vi "CryoServer GUI.vi"(9 "Standalone":bool=TRUE, 10 "Init Data":variant, 11 "Filter Wheel name":string) -> ()   [LabVIEW 2021]
uses:
  CryoServer cluster Settings.ctl
  CryoServer.lvclass
  CryoServer Telemetry Map.ctl
  Subsystems/SS typedef cluster Instrument Command Queue Data.ctl
  Subsystems/SS cluster Data Queue type.ctl
  CryoServer Channel Mapping.ctl
  hk-channel-class/HK Item/HK Channel cluster Telemetry Data.ctl
  hk-channel-class/HK Item/HK Channel enum Data Type.ctl
  <vilib>/Utility/error.llb/DialogType.ctl
  typedefs/CC cluster Alarm Data.ctl
  <vilib>/Analysis/baseanly.llb/Mean (DBL).vi
  hk-channel-class/HK Item/HK Item.lvclass
  <vilib>/Analysis/NI_AALBase.lvlib
panel:
  in  "Settings":bool
  in  "System Health":bool
  in  "HK Window":bool
  in  "Close":bool
  in  "Re-connect":bool
  in  "IP Address":string
  out "Response":string
  in  "Send":bool
  in  "Piper Board ID (Hex)":u32=10 format="%02x"
  in  "Piper Command":string
  out "Connected?":bool
  in  "Temperatures Values":i32[](listbox)
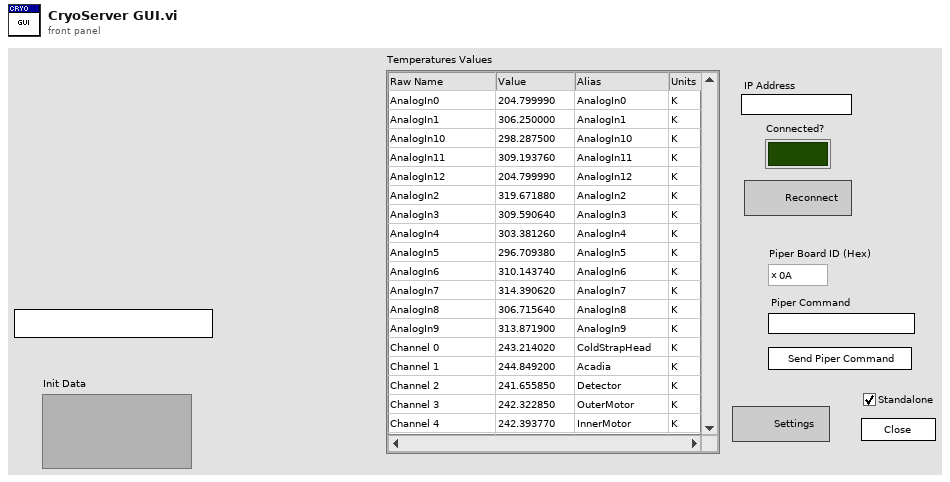
[diagram p1: front panel]
types:
  T1 = typedef "CryoServer cluster Settings.ctl" = cluster{"Address":string}
  T2 = typedef "CryoServer Telemetry Map.ctl" = map{string, dbl[]}
  T3 = typedef "SS typedef cluster Instrument Command Queue Data.ctl" = cluster{"Cmd":string, "Parameters":variant}
  T4 = typedef "CryoServer Channel Mapping.ctl" = cluster{"Alias":string, "Units":string}
  T5 = cluster{"state":refnum<user-event>, "Settings":T1, "CryoServer":refnum<class "CryoServer.lvclass">, "Telem":T2, "cntrl q":refnum<queue>, "Data Q":refnum<queue>, "Ch Names":string[], "Values":dbl[], "Cmd":T3, "Next Poll":timestamp, "error":errorcluster, "Ch Map":map{string, T4}, "Setting VI":refnum<vi>}
  T6 = typedef "SS cluster Data Queue type.ctl" = cluster{"Source":string, "Type":string, "Data":variant}
  T7 = typedef "HK Item.lvclass/HK Channel enum Data Type.ctl" = enum16{"Floating Point", "Integer", "Enum", "String", "Waveform", "File"}
  T8 = typedef "HK Item.lvclass/HK Channel cluster Telemetry Data.ctl" = cluster{"Ch Names":string[], "Ch Values":dbl[], "Timestamp":timestamp, "Data Type":T7}
  T9 = typedef "CC cluster Alarm Data.ctl" = cluster{"Measured Value":dbl, "Alarm Low":dbl, "Alarm High":dbl, "Message":string, "Source":string}
  T10 = typedef "DialogType.ctl" = u16
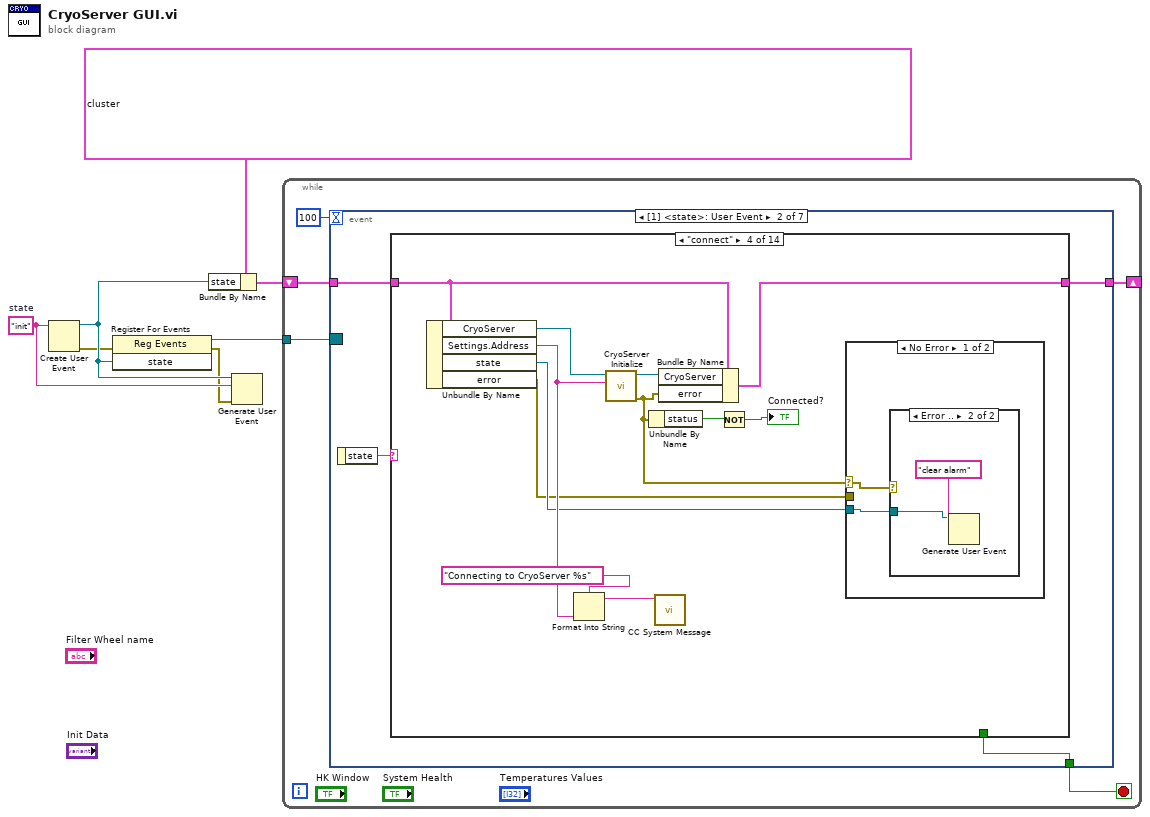
[diagram p0: block diagram]
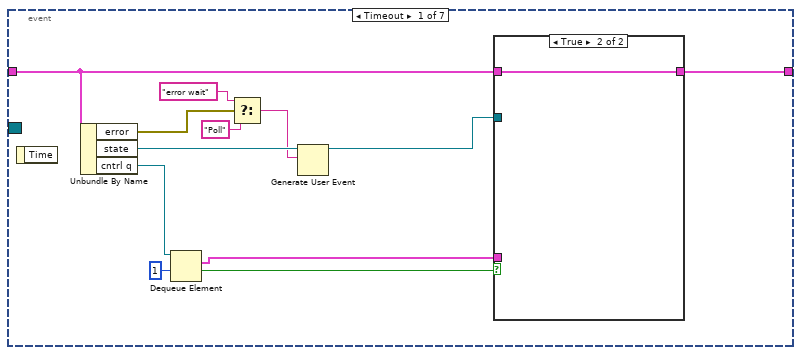
[diagram p2: hidden frame]
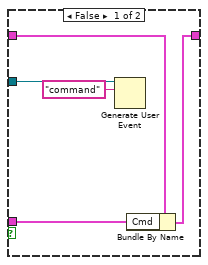
[diagram p3: hidden frame]
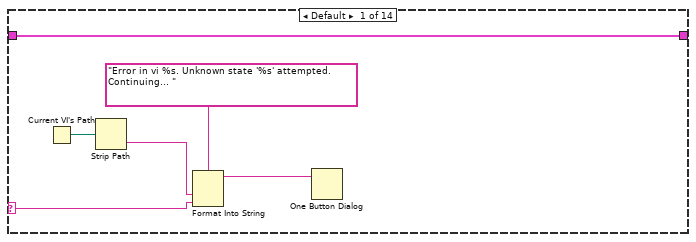
[diagram p4: hidden frame]
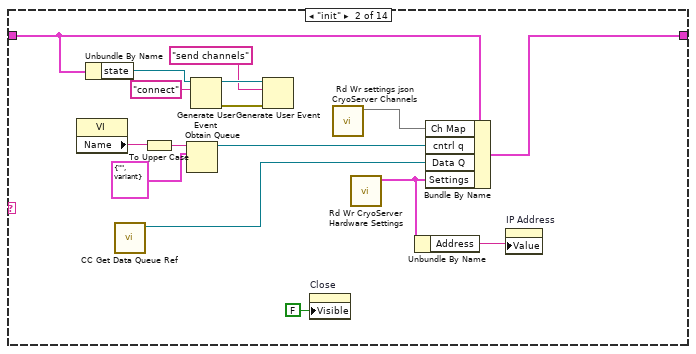
[diagram p5: hidden frame]
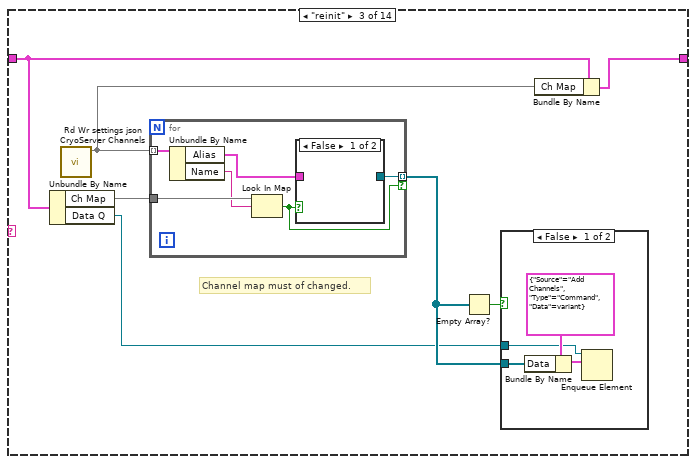
[diagram p6: hidden frame]
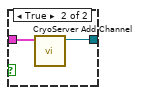
[diagram p8: hidden frame]
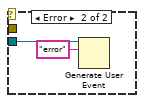
[diagram p10: hidden frame]
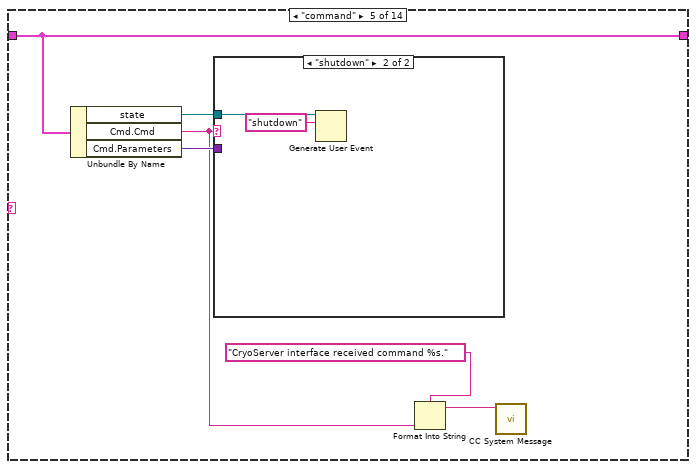
[diagram p11: hidden frame]
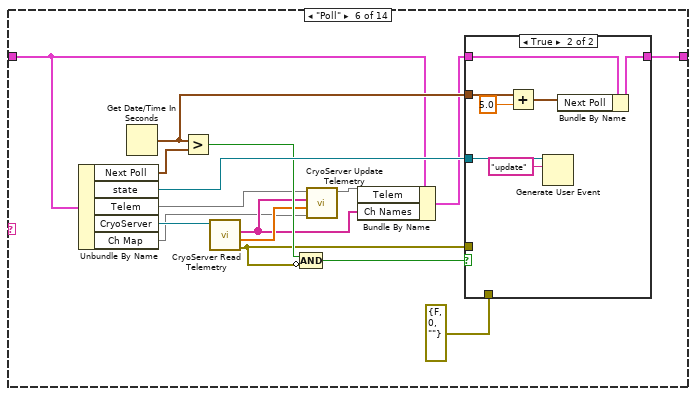
[diagram p13: hidden frame]
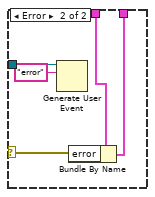
[diagram p15: hidden frame]
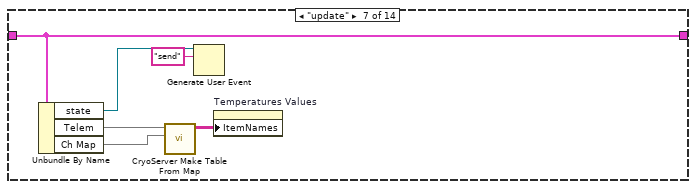
[diagram p16: hidden frame]
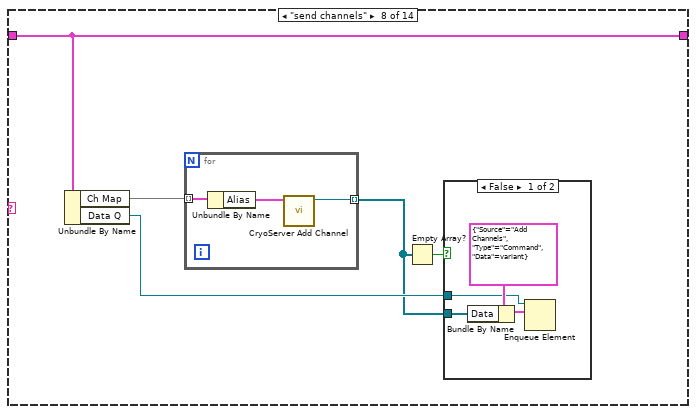
[diagram p17: hidden frame]
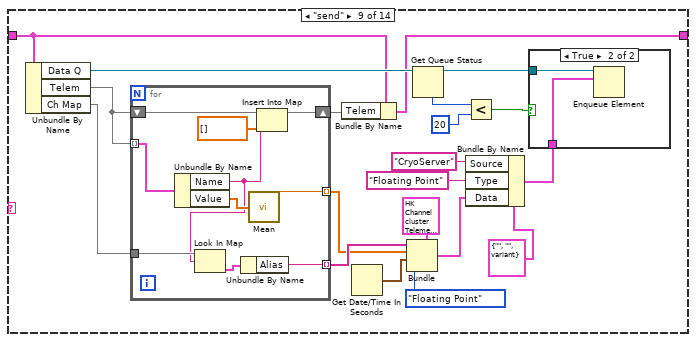
[diagram p19: hidden frame]
diagram:
  w3 = "init"  # state
  n1 = Create User Event(user event datatype=w3) -> (user event=w5:refnum<user-event>, error out=w1:errorcluster)  [unwired: 1 in]
  n2 = register-events(error in=w1, w5) -> (reference out=w4:refnum<event-registration>, error out=w2:errorcluster)  [unwired: 1 in]
  n3 = Bundle By Name(cluster=T5 {"state"=refnum, "Settings"={"Address"=""}, "CryoServer"=refnum, "Telem"={}, "cntrl q"=refnum, "Data Q"=refnum, "Ch Names"=[], "Values"=[], "Cmd"={"Cmd"="", "Parameters"=variant}, "Next Poll"=timestamp(0 s since 1904-01-01), "error"={"status"=FALSE, "code"=0, "source"=""}, "Ch Map"={}, "Setting VI"=refnum}, "state"=w5) -> (w6:T5)
  n4 = Generate User Event(user event=w5, event data cluster=w3, error in=w2) -> ()  [unwired: 1 in, 2 out]
  n5 = while {
    tunnel: w4 -> [w12]
    shift-right: [w10] -> _
    shift-left: w6 -> [w11]
    stop <- w9 stop-if-true
    n6 = event shown="[1] <state>: User Event" {
      selector: w12 -> [_ _ _ _ _ _ _]
      dyn-events: _ -> [_ _ _ _ _ _ _]
      timeout: 100 -> [_ _ _ _ _ _ _]
      tunnel: w11 -> [w17 w33 w239 w240 w251 w258 w261]
      tunnel: [w20 w32 w239 w241 w252 w258 w261] -> w10
      tunnel: [_ w31 _ _ _ _ _] -> w9
      event Timeout {
        n7 = event-data() -> ()  [unwired: 1 in, 1 out]
        n8 = Unbundle By Name(w17) -> ("error"=w16:errorcluster, "state"=w19:refnum<user-event>, "cntrl q"=w24:refnum<queue>)
        n9 = Dequeue Element(queue=w24, timeout in ms (-1)=1) -> (element=w21:T3, timed out?=w22:bool)  [unwired: 1 in, 2 out]
        n10 = Select(t="error wait" ("event data"), s=w16, f="Poll" ("event data")) -> (s? t:f=w13:string)
        n11 = Generate User Event(user event=w19, event data cluster=w13) -> (user event out=w18:refnum<user-event>)  [unwired: 2 in, 1 out]
        n12 = case shown="True" w22 {
          tunnel: w17 -> [w29 w30]
          tunnel: w21 -> [w28 _]
          tunnel: w18 -> [w27 _]
          tunnel: [w25 w30] -> w20
          frame False {
            n13 = Generate User Event(user event=w27, event data cluster="command" ("event data")) -> ()  [unwired: 2 in, 2 out]
            n14 = Bundle By Name(cluster=w29, "Cmd"=w28) -> (w25:T5)
          }
          frame True {
          }
        }
      }
      event User Event {
        n15 = event-data() -> ("state"=w34:string)  [unwired: 1 in]
        n16 = case shown="\"connect\"" w34 {
          selector: w34 -> [w39 _ _ _ _ _ _ _ _ _ _ _ _ _]
          tunnel: w33 -> [w35 w53 w62 w85 w99 w108 w138 w141 w154 w189 w194 w216 w219 w232]
          tunnel: [w35 w56 w63 w77 w99 w115 w138 w141 w155 w189 w199 w216 w219 w232] -> w32
          tunnel: [_ _ _ _ _ _ _ _ _ _ _ _ _ TRUE] -> w31
          frame Default {
            n17 = Current VI's Path() -> (path=w38:path)
            n18 = Strip Path(path=w38) -> (name=w37:string)  [unwired: 1 out]
            n19 = Format Into String(format string="Error in vi %s. Unknown state '%s' attempted. Continuing... ", w37, w39) -> (resulting string=w36:string)  [unwired: 2 in, 1 out]
            n20 = One Button Dialog(message=w36) -> ()  [unwired: 1 in, 1 out]
          }
          frame "init" {
            n21 = property class="VI"() -> ("Name"=w50:string)  [unwired: 2 in, 2 out]
            n22 = Unbundle By Name(w53) -> ("state"=w52:refnum<user-event>)
            n23 = call "CC Get Data Queue Ref.vi"() -> ("Data Q"=w46:refnum<queue>)  [unwired: 10 in, 1 out]
            n24 = To Upper Case(1:w50) -> (0:w49:string)
            n25 = Obtain Queue(name (unnamed)=w49, element data type=T3 {"Cmd"="", "Parameters"=variant}) -> (queue out=w47:refnum<queue>)  [unwired: 3 in, 2 out]
            n26 = Generate User Event(user event=w52, event data cluster="connect" ("event data")) -> (user event out=w44:refnum<user-event>, error out=w43:errorcluster)  [unwired: 2 in]
            n27 = Generate User Event(user event=w44, event data cluster="send channels" ("event data"), error in=w43) -> ()  [unwired: 1 in, 2 out]
            n28 = property on="Close" class="Bool"("Visible"=FALSE) -> ()  [unwired: 2 in, 2 out]
            n29 = call "Rd Wr settings json CryoServer Channels.vi"() -> ("CryoServer Channels out"=w45:map{string, T4})  [unwired: 9 in, 2 out]
            n30 = call "Rd Wr CryoServer Hardware Settings.vi"() -> ("CryoServer Settings"=w55:T1)  [unwired: 10 in, 1 out]
            n31 = Unbundle By Name(w55) -> ("Address"=w54:string)
            n32 = Bundle By Name(cluster=w53, "Ch Map"=w45, "cntrl q"=w47, "Data Q"=w46, "Settings"=w55) -> (w56:T5)
            n33 = property on="IP Address" class="Str"("Value"=w54) -> ()  [unwired: 2 in, 2 out]
          }
          frame "reinit" {
            # "Channel map must of changed."
            n34 = Unbundle By Name(w62) -> ("Ch Map"=w60:map{string, T4}, "Data Q"=w57:refnum<queue>)
            n35 = call "Rd Wr settings json CryoServer Channels.vi"() -> ("CryoServer Channels out"=w61:map{string, T4})  [unwired: 9 in, 2 out]
            n36 = for {
              tunnel: w61 -> [w72] mode=indexing
              tunnel: w60 -> [w73]
              tunnel: [w69] -> w58 mode=indexing if=w68
              n37 = Unbundle By Name(w72) -> ("Alias"=w70:T4, "Name"=w71:string)
              n38 = Look In Map(map=w73, key=w71) -> (key not found?=w68:bool)  [unwired: 1 in, 1 out]
              n39 = case shown="False" w68 {
                tunnel: w70 -> [_ w75]
                tunnel: [_ w74] -> w69
                frame False {
                }
                frame True {
                  n40 = call "CryoServer Add Channel.vi"("value"=w75) -> ("HK Item out"=w74:refnum<class "HK Item.lvclass">)  [unwired: 10 in]
                }
              }
            }
            n41 = Empty Array?(array=w58) -> (empty?=w59:bool)
            n42 = case shown="False" w59 {
              tunnel: w57 -> [w65 _]
              tunnel: w58 -> [w64 _]
              frame False {
                n43 = Bundle By Name(cluster=T6 {"Source"="Add Channels", "Type"="Command", "Data"=variant} ("element"), "Data"=w64) -> (w67:T6)
                n44 = Enqueue Element(queue=w65, element=w67) -> ()  [unwired: 2 in, 3 out]
              }
              frame True {
              }
            }
            n45 = Bundle By Name(cluster=w62, "Ch Map"=w61) -> (w63:T5)
          }
          frame "connect" {
            n46 = Unbundle By Name(w85) -> ("CryoServer"=w87:refnum<class "CryoServer.lvclass">, "Settings.Address"=w80:string, "state"=w78:refnum<user-event>, "error"=w76:errorcluster)
            n47 = Format Into String(format string="Connecting to CryoServer %s" ("Message"), w80) -> (resulting string=w81:string)  [unwired: 2 in, 1 out]
            n48 = call-dynamic "CryoServer Initialize.vi"("address"=w80, "CryoServer in"=w87) -> ("error out"=w79:errorcluster, "CryoServer out"=w86:refnum<class "CryoServer.lvclass">)  [unwired: 8 in]
            n49 = Unbundle By Name(w79) -> ("status"=w84:bool)
            n50 = call "CC System Message.vi"("Message"=w81) -> ()  [unwired: 10 in, 1 out]
            n51 = Bundle By Name(cluster=w85, "CryoServer"=w86, "error"=w79) -> (w77:T5)
            n52 = Not(x=w84) -> (.not. x?=→"Connected?":bool)
            n53 = case shown="No Error" w79 {
              selector: w79 -> [w89 _]
              tunnel: w78 -> [w88 w93]
              tunnel: w76 -> [_ _]
              frame No Error {
                n54 = case shown="Error .." w89 {
                  tunnel: w88 -> [_ w90]
                  frame No Error {
                  }
                  frame Error {
                    n55 = Generate User Event(user event=w90, event data cluster="clear alarm" ("event data")) -> ()  [unwired: 2 in, 2 out]
                  }
                }
              }
              frame Error {
                n56 = Generate User Event(user event=w93, event data cluster="error" ("event data")) -> ()  [unwired: 2 in, 2 out]
              }
            }
          }
          frame "command" {
            n57 = Unbundle By Name(w99) -> ("state"=w98:refnum<user-event>, "Cmd.Cmd"=w94:string, "Cmd.Parameters"=w97:variant)
            n58 = case shown="\"shutdown\"" w94 {
              tunnel: w98 -> [_ w101]
              tunnel: w97 -> [_ _]
              frame "False", Default {
              }
              frame "shutdown" {
                n59 = Generate User Event(user event=w101, event data cluster="shutdown" ("event data")) -> ()  [unwired: 2 in, 2 out]
              }
            }
            n60 = Format Into String(format string="CryoServer interface received command %s." ("Message"), w94) -> (resulting string=w95:string)  [unwired: 2 in, 1 out]
            n61 = call "CC System Message.vi"("Message"=w95) -> ()  [unwired: 10 in, 1 out]
          }
          frame "Poll" {
            n62 = Unbundle By Name(w108) -> ("Next Poll"=w114:timestamp, "state"=w116:refnum<user-event>, "Telem"=w110:T2, "CryoServer"=w117:refnum<class "CryoServer.lvclass">, "Ch Map"=w104:map{string, T4})
            n63 = Get Date/Time In Seconds() -> (seconds since 1Jan1904=w113:timestamp)
            n64 = Greater?(x=w113, y=w114) -> (0:w112:bool)
            n65 = call-dynamic "CryoServer Read Telemetry.vi"("CryoServer in"=w117) -> ("error out"=w103:errorcluster, "Values"=w109:dbl[], "Ch Names"=w105:string[])  [unwired: 5 in, 3 out]
            n66 = Compound Arithmetic op=AND(w112, invert w103) -> (w111:bool)
            n67 = call "CryoServer Update Telemetry.vi"("CryoServer Channels"=w104, "Values"=w109, "Ch Names"=w105, "Telem"=w110) -> ("Telem out"=w106:T2)  [unwired: 7 in]
            n68 = Bundle By Name(cluster=w108, "Telem"=w106, "Ch Names"=w105) -> (w107:T5)
            n69 = case shown="True" w111 {
              tunnel: w107 -> [w119 w134]
              tunnel: [w120 w133] -> w115
              tunnel: w116 -> [w121 w132]
              tunnel: w113 -> [_ w129]
              tunnel: w103 -> [_ _]
              tunnel: errorcluster {"status"=FALSE, "code"=0, "source"=""} ("error out") -> [w118 _]
              frame False {
                n70 = case shown="No Error" w118 {
                  selector: w118 -> [_ w124]
                  tunnel: w121 -> [_ w127]
                  tunnel: w119 -> [w122 w125]
                  tunnel: [w122 w123] -> w120
                  frame No Error {
                  }
                  frame Error {
                    n71 = Generate User Event(user event=w127, event data cluster="error" ("event data")) -> ()  [unwired: 2 in, 2 out]
                    n72 = Bundle By Name(cluster=w125, "error"=w124) -> (w123:T5)
                  }
                }
              }
              frame True {
                n73 = Add(x=w129, y=5.0) -> (x+y=w128:timestamp)
                n74 = Generate User Event(user event=w132, event data cluster="update" ("event data")) -> ()  [unwired: 2 in, 2 out]
                n75 = Bundle By Name(cluster=w134, "Next Poll"=w128) -> (w133:T5)
              }
            }
          }
          frame "update" {
            n76 = Unbundle By Name(w138) -> ("state"=w140:refnum<user-event>, "Telem"=w136:T2, "Ch Map"=w135:map{string, T4})
            n77 = call "CryoServer Make Table From Map.vi"("Ch Map"=w135, "Telem"=w136) -> ("table"=w137:string[][])  [unwired: 9 in]
            n78 = Generate User Event(user event=w140, event data cluster="send" ("event data")) -> ()  [unwired: 2 in, 2 out]
            n79 = property on="Temperatures Values" class="MCListbox (strict)"("ItemNames"=w137) -> ()  [unwired: 2 in, 2 out]
          }
          frame "send channels" {
            n80 = Unbundle By Name(w141) -> ("Ch Map"=w142:map{string, T4}, "Data Q"=w145:refnum<queue>)
            n81 = for {
              tunnel: [w152] -> w144 mode=indexing
              tunnel: w142 -> [w151] mode=indexing
              n82 = Unbundle By Name(w151) -> ("Alias"=w150:T4)
              n83 = call "CryoServer Add Channel.vi"("value"=w150) -> ("HK Item out"=w152:refnum<class "HK Item.lvclass">)  [unwired: 10 in]
            }
            n84 = Empty Array?(array=w144) -> (empty?=w143:bool)
            n85 = case shown="False" w143 {
              tunnel: w145 -> [w147 _]
              tunnel: w144 -> [w146 _]
              frame False {
                n86 = Bundle By Name(cluster=T6 {"Source"="Add Channels", "Type"="Command", "Data"=variant} ("element"), "Data"=w146) -> (w149:T6)
                n87 = Enqueue Element(queue=w147, element=w149) -> ()  [unwired: 2 in, 3 out]
              }
              frame True {
              }
            }
          }
          frame "send" {
            n88 = Unbundle By Name(w154) -> ("Data Q"=w162:refnum<queue>, "Telem"=w157:T2, "Ch Map"=w153:map{string, T4})
            n89 = for {
              tunnel: w157 -> [w184] mode=indexing
              tunnel: [w175] -> w167 mode=indexing
              tunnel: [w182] -> w166 mode=indexing
              shift-right: [w179] -> w156
              shift-left: w157 -> [w181]
              tunnel: w153 -> [w178]
              n90 = Unbundle By Name(w184) -> ("Name"=w177:string, "Value"=w183:dbl[])
              n91 = Look In Map(map=w178, key=w177) -> (value=w176:T4)  [unwired: 1 in, 1 out]
              n92 = Unbundle By Name(w176) -> ("Alias"=w175:string)
              n93 = call-poly <vilib>:"Mean.vi"("X"=w183) -> ("mean"=w182:dbl)  [unwired: 1 out]
              n94 = Insert Into Map(map in=w181, key=w177, value=dbl[] []) -> (map out=w179:T2)  [unwired: 2 out]
            }
            n95 = Bundle By Name(cluster=w154, "Telem"=w156) -> (w155:T5)
            n96 = Get Date/Time In Seconds() -> (seconds since 1Jan1904=w165:timestamp)
            n97 = Bundle(cluster=T8 {"Ch Names"=[], "Ch Values"=[], "Timestamp"=timestamp(0 s since 1904-01-01), "Data Type"=enum."Floating Point"}, "Ch Names"=w167, "Ch Values"=w166, "Timestamp"=w165, "Data Type"=HK_Channel_enum_Data_Type."Floating Point") -> (w169:T8)
            n98 = Get Queue Status(queue=w162) -> (queue out=w161:refnum<queue>, # elements in queue=w160:i32)  [unwired: 2 in, 6 out]
            n99 = Less?(x=w160, y=20) -> (x < y?=w158:bool)
            n100 = Bundle By Name(cluster=T6 {"Source"="", "Type"="", "Data"=variant} ("element"), "Source"="CryoServer", "Type"="Floating Point" ("Data Type"), "Data"=w169) -> (w163:T6)
            n101 = case shown="True" w158 {
              tunnel: w163 -> [_ w174]
              tunnel: w161 -> [_ w173]
              frame False {
                # "If Q is filling up, don't send. This VI is probably running standalone"
              }
              frame True {
                n102 = Enqueue Element(queue=w173, element=w174) -> ()  [unwired: 2 in, 3 out]
              }
            }
          }
          frame "piper command" {
            n103 = Unbundle By Name(w189) -> ("CryoServer"=w188:refnum<class "CryoServer.lvclass">)
            n104 = call-dynamic "CryoServer Send Piper Passthrough.vi"("Piper Command"="Piper Command", "Piper Board ID (Hex)"="Piper Board ID (Hex)", "CryoServer in"=w188) -> ("Response"=→"Response":string)  [unwired: 6 in, 2 out]
          }
          frame "error" {
            w191 = "CryoServer" ("Source")
            w205 = T10 0 items=["no dialog", "OK message", "continue or stop message", "OK message + warnings", "continue/stop + warnings"] ("type of dialog (OK msg:1)")
            n105 = Unbundle By Name(w194) -> ("error"=w208:errorcluster, "error.code"=w211:i32, "error.source"=w209:string)
            n106 = Unbundle By Name(w194) -> ("Data Q"=w198:refnum<queue>)
            n107 = local write "Connected?"(FALSE ("Connected?")) -> ()
            n108 = Bundle By Name(cluster=T9 {"Measured Value"=0.0, "Alarm Low"=0.0, "Alarm High"=0.0, "Message"="", "Source"=""} ("element"), "Source"=w191, "Message"="CryoCooler Comminications Error") -> (w192:T9)
            n109 = call <vilib>:"Simple Error Handler.vi"("type of dialog (OK msg:1)"=w205, "error in (no error)"=w208) -> ("message"=w207:string)  [unwired: 3 in, 4 out]
            n110 = Bundle By Name(cluster=T6 {"Source"="", "Type"="", "Data"=variant} ("element"), "Source"=w191, "Type"="Alarm Set", "Data"=w192) -> (w195:T6)
            n111 = Get Date/Time In Seconds() -> (seconds since 1Jan1904=w202:timestamp)
            n112 = Add(x=w202, y=300.0) -> (x+y=w200:timestamp)
            n113 = Format Into String(format string="Error from %s. Error # %d, Error Source: %s, Error message \"%s\"", "CryoServer" ("input 1"), w211, w209, w207) -> (resulting string=w206:string)  [unwired: 2 in, 1 out]
            n114 = Enqueue Element(queue=w198, element=w195) -> ()  [unwired: 2 in, 3 out]
            n115 = Bundle By Name(cluster=w194, "Next Poll"=w200) -> (w199:T5)
            n116 = call "CryoCooler Message Log.vi"("String in"=w206) -> ()  [unwired: 9 in, 2 out]
          }
          frame "error wait" {
            n117 = Unbundle By Name(w216) -> ("Next Poll"=w213:timestamp, "state"=w212:refnum<user-event>)
            n118 = Get Date/Time In Seconds() -> (seconds since 1Jan1904=w215:timestamp)
            n119 = Greater?(x=w215, y=w213) -> (0:w214:bool)
            n120 = case shown="False" w214 {
              tunnel: w213 -> [_ _]
              tunnel: w212 -> [_ w218]
              frame False {
              }
              frame True {
                n121 = Generate User Event(user event=w218, event data cluster="connect" ("event data")) -> ()  [unwired: 2 in, 2 out]
              }
            }
          }
          frame "clear alarm" {
            w221 = "CryoServer" ("Source")
            n122 = Unbundle By Name(w219) -> ("Data Q"=w227:refnum<queue>)
            n123 = Bundle By Name(cluster=T9 {"Measured Value"=0.0, "Alarm Low"=0.0, "Alarm High"=0.0, "Message"="", "Source"=""} ("element"), "Source"=w221, "Message"="CryoCooler Comminications Error") -> (w222:T9)
            n124 = Bundle By Name(cluster=T6 {"Source"="", "Type"="", "Data"=variant} ("element"), "Source"=w221, "Type"="Alarm Clear", "Data"=w222) -> (w224:T6)
            n125 = Enqueue Element(queue=w227, element=w224) -> ()  [unwired: 2 in, 3 out]
          }
          frame "shutdown" {
            n126 = Unbundle By Name(w232) -> ("Setting VI"=w228:refnum<vi>, "CryoServer"=w231:refnum<class "CryoServer.lvclass">)
            n127 = call-dynamic "CryoServer Close.vi"("CryoServer in"=w231) -> ()  [unwired: 9 in, 2 out]
            n128 = Not A Number/Path/Refnum?(number/path/refnum=w228) -> (NaN/Path/Refnum?=w229:bool)
            n129 = case shown="True" w229 {
              tunnel: w228 -> [_ w237]
              frame False {
              }
              frame True {
                n130 = invoke class="VI (strict)" method="Abort VI"(reference=w237) -> (reference out=w234:refnum<vi>, error out=w236:errorcluster)  [unwired: 2 in, 1 out]
                n131 = call <vilib>:"Clear Errors.vi"("error in (no error)"=w236) -> ("error out"=w235:errorcluster)  [unwired: 5 in, 1 out]
                n132 = Close Reference(reference=w234, error in (no error)=w235) -> (error out=w233:errorcluster)
                n133 = call <vilib>:"Clear Errors.vi"("error in (no error)"=w233) -> ()  [unwired: 5 in, 2 out]
              }
            }
          }
        }
      }
      event "Standalone": Value Change {
        n134 = event-data() -> ()  [unwired: 1 in, 6 out]
        n135 = property on="Close" class="Bool"("Visible"="Standalone") -> ()  [unwired: 2 in, 2 out]
      }
      event "Settings": Value Change {
        n136 = event-data() -> ()  [unwired: 1 in, 6 out]
        n137 = vi-ref "CryoServer Configure.vi"() -> (w249:refnum<vi>)
        n138 = property class="VI Interface Type 2"(reference=w249) -> (reference out=w245:refnum<vi>, "Path"=w248:path)  [unwired: 1 in, 1 out]
        n139 = Unbundle By Name(w240) -> ("Ch Names"=w244:string[], "cntrl q"=w243:refnum<queue>)
        n140 = Open VI Reference(type specifier VI Refnum (for type only)=w245, vi path=w248, options=128) -> (vi reference=w246:refnum<vi>)  [unwired: 3 in, 1 out]
        n141 = call-by-ref "Start Asynchronous Call"(reference=w246, "cntrl q"=w243, "Ch Names"=w244) -> (reference out=w242:refnum<vi>)  [unwired: 10 in, 2 out]
        n142 = Bundle By Name(cluster=w240, "Setting VI"=w242) -> (w241:T5)
      }
      event "Re-connect": Value Change {
        n143 = event-data() -> ()  [unwired: 1 in, 6 out]
        n144 = Unbundle By Name(w251) -> ("CryoServer"=w250:refnum<class "CryoServer.lvclass">, "state"=w255:refnum<user-event>)
        n145 = Generate User Event(user event=w255, event data cluster="connect" ("event data")) -> ()  [unwired: 2 in, 2 out]
        n146 = call-dynamic "CryoServer Close.vi"("CryoServer in"=w250) -> ()  [unwired: 9 in, 2 out]
        n147 = Bundle By Name(cluster=w251, "Settings.Address"="IP Address") -> (w252:T5)
      }
      event "Send": Value Change {
        n148 = event-data() -> ()  [unwired: 1 in, 6 out]
        n149 = Unbundle By Name(w258) -> ("state"=w257:refnum<user-event>)
        n150 = Generate User Event(user event=w257, event data cluster="piper command" ("event data")) -> ()  [unwired: 2 in, 2 out]
      }
      event "Close": Value Change {
        n151 = event-data() -> ()  [unwired: 1 in, 2 out]
        n152 = Unbundle By Name(w261) -> ("state"=w260:refnum<user-event>)
        n153 = Generate User Event(user event=w260, event data cluster="shutdown" ("event data")) -> ()  [unwired: 2 in, 2 out]
      }
    }
  }
